vi "RGB WS2812 Control VI_DYLAN_DONE0312_Computertime.vi"() -> ()   [LabVIEW 2019]
uses:
  VI States.ctl
  <vilib>/Instr/_visa.llb/VISA Configure Serial Port (Instr).vi
  <vilib>/MakerHub/LINX/LMH-LINX.lvlib
panel:
  in  "OK Button":bool
  in  "RED 3":dbl(slide) scale=0.0..250.0
  out "RED 4":dbl format="%#_3g"
  in  "?":dbl(slide) scale=0.0..250.0
  out "?":dbl format="%#_3g"
  in  "OK Button 2":bool
  in  "Black [s]":i32
  in  "Blue [s]":i32
  in  "Red [s]":u32
  out "BlueLED":bool
  out "RedLED":bool
  out "Current date string":string
  out "Current time string":string
  out "Start light":bool
  in  "Set time x:xx AM format 2":string="8:55 AM"
  in  "VISA resource name":refnum<visa-resource-name>
  in  "Stop Button":bool
  out "Loop \nRate (Hz)":u32
  out "LeftY 2":i32
  out "LeftX 2":i32
  in  "To 1st left = dont touch":dbl format="%#_13g"
  in  "Set time x:xx AM format":string="8:55 AM"
  out "x = y?":bool
  out "time string":string
  out "date string":string
  in  "stop 2":bool
  out "Walking":bool
  in  "GO":bool
  out "RightY":i32
  out "LeftY":i32
  out "RightX":i32
  out "LeftX":i32
  in  "Repeats":i32
  in  "To Right [s]":dbl format="%#_13g"
  in  "To Left[s]":dbl format="%#_13g"
  in  "PyModule for Python 3.7":path=path "C:/Users/xwghu/Desktop/AutoControlKit/mouseControl.py"
  out "?":refnum<k35>
  in  "Python version":string="3.7"
  # "Mouse control"
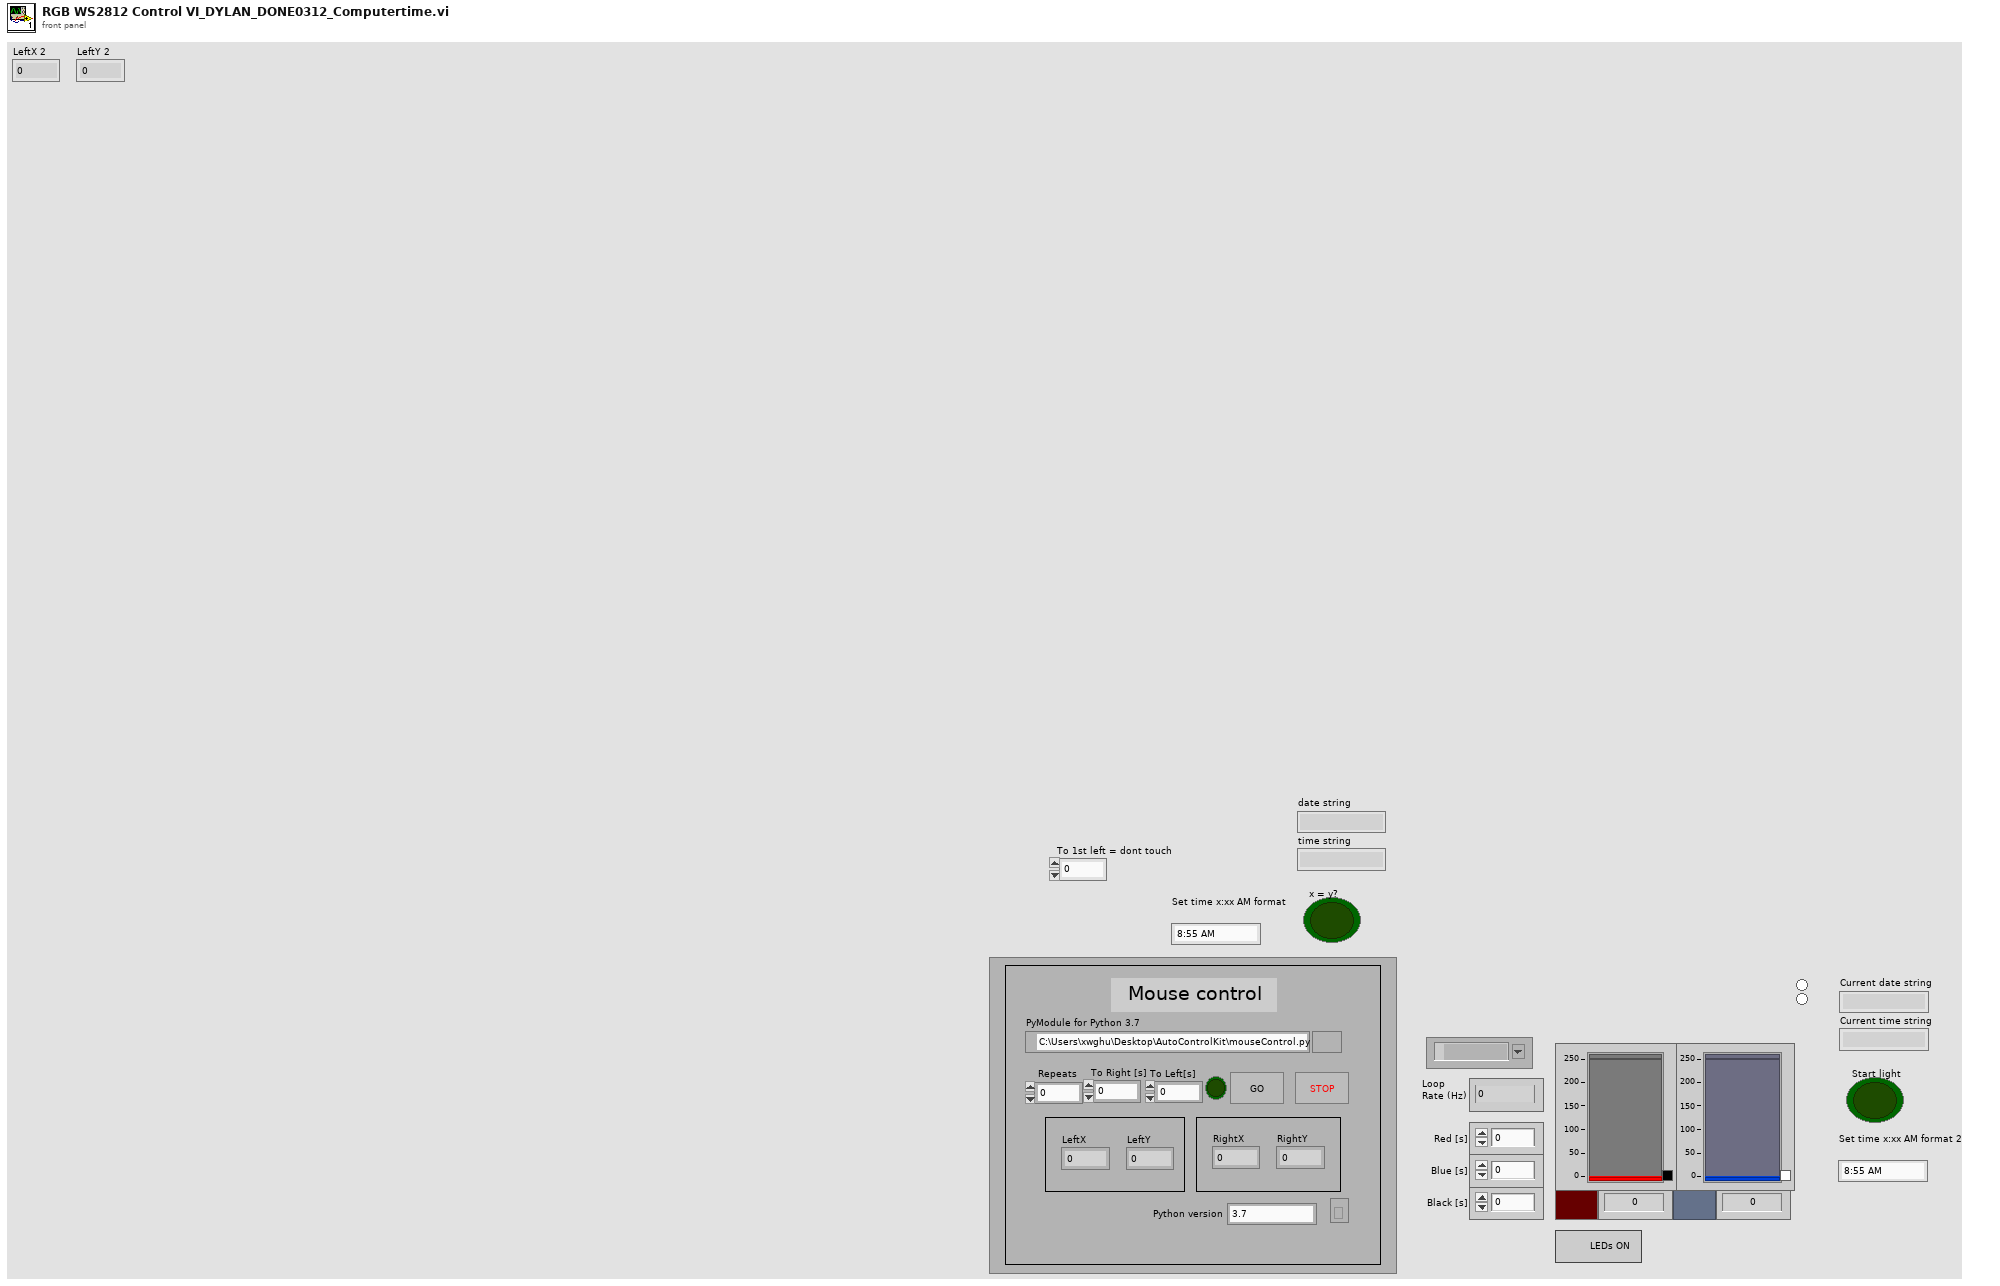
[diagram p1: front panel]
types:
  T1 = typedef "VI States.ctl" = enum16{"Poll", "Init Serial", "Read Serial", "Acq Sound", "Close Serial"}
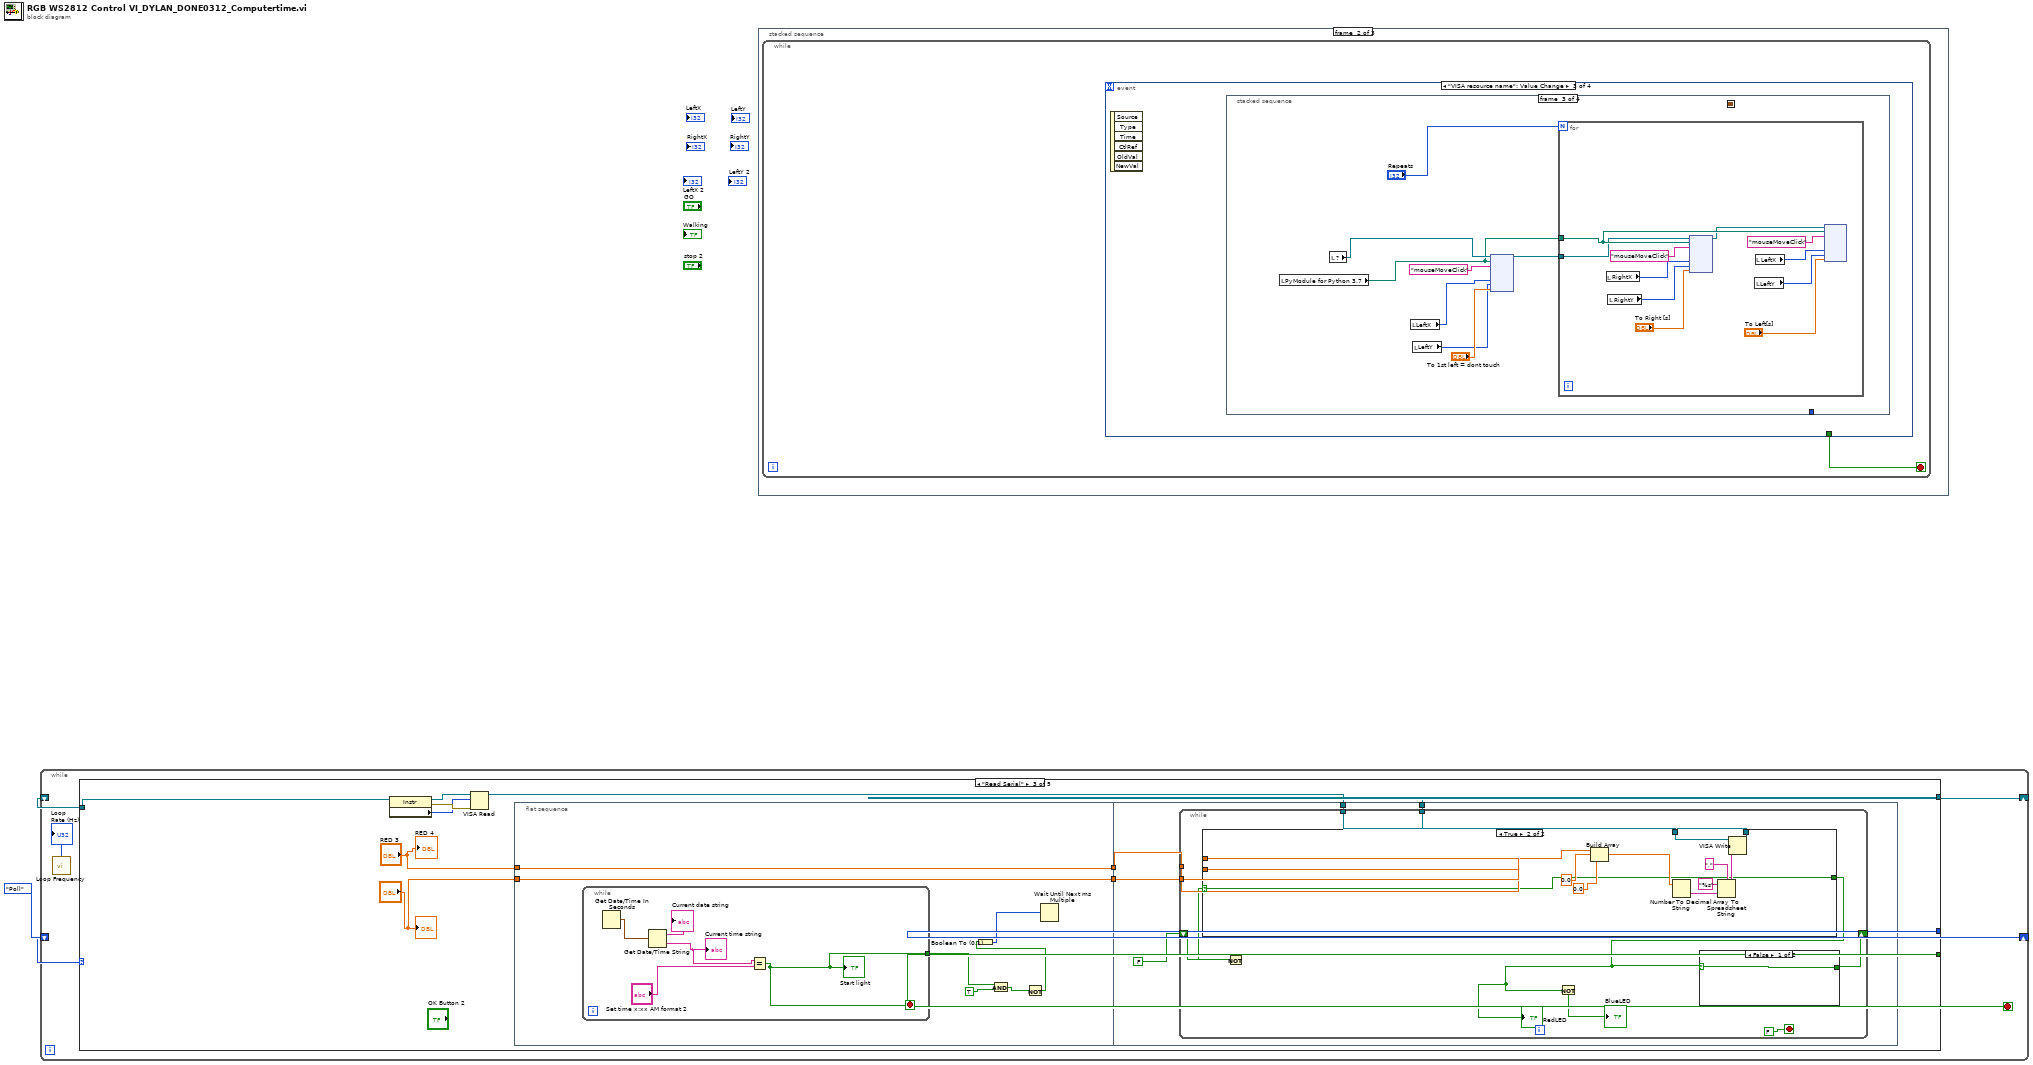
[diagram p0: block diagram]
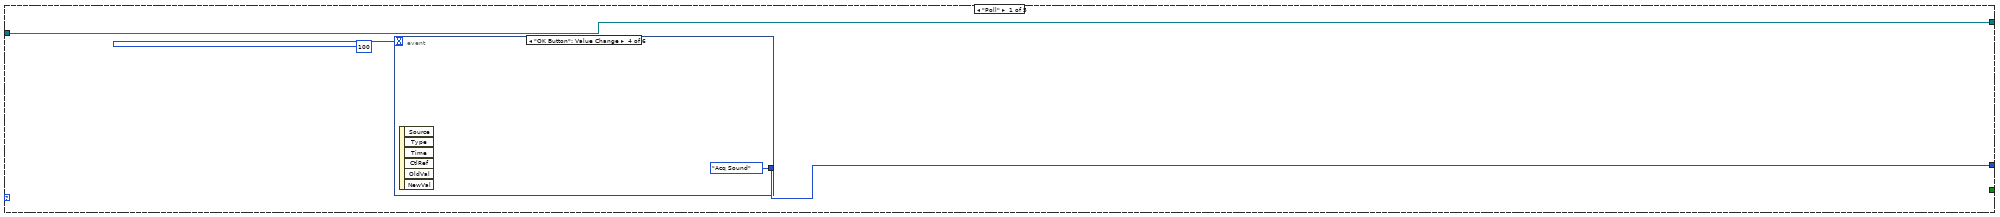
[diagram p2: hidden frame]
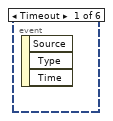
[diagram p3: hidden frame]
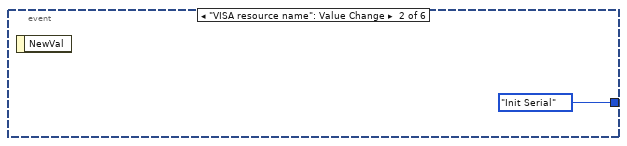
[diagram p4: hidden frame]
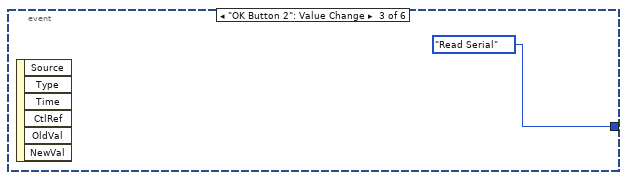
[diagram p5: hidden frame]
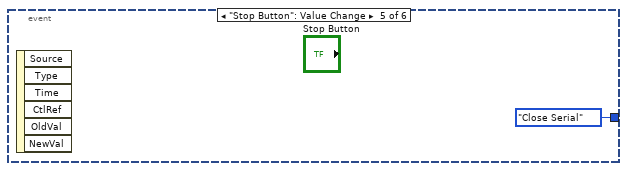
[diagram p6: hidden frame]
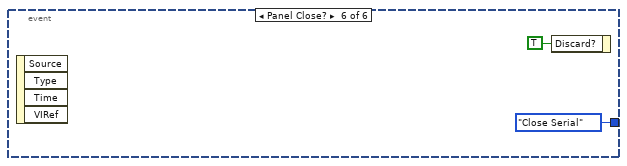
[diagram p7: hidden frame]
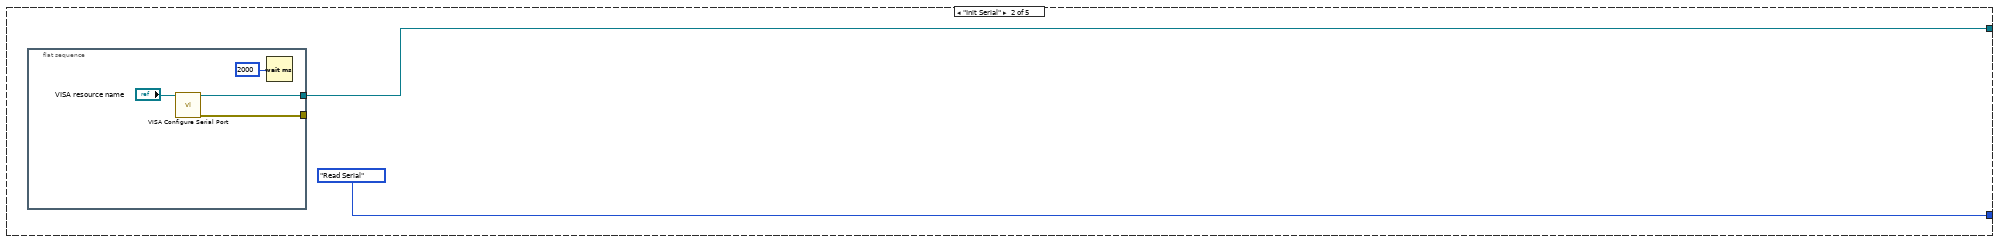
[diagram p8: hidden frame]
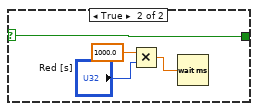
[diagram p9: hidden frame]
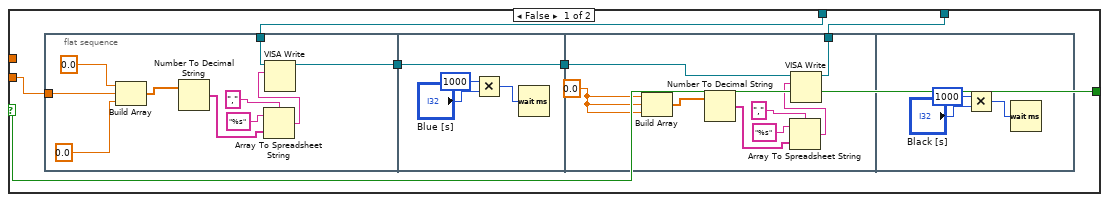
[diagram p10: hidden frame]
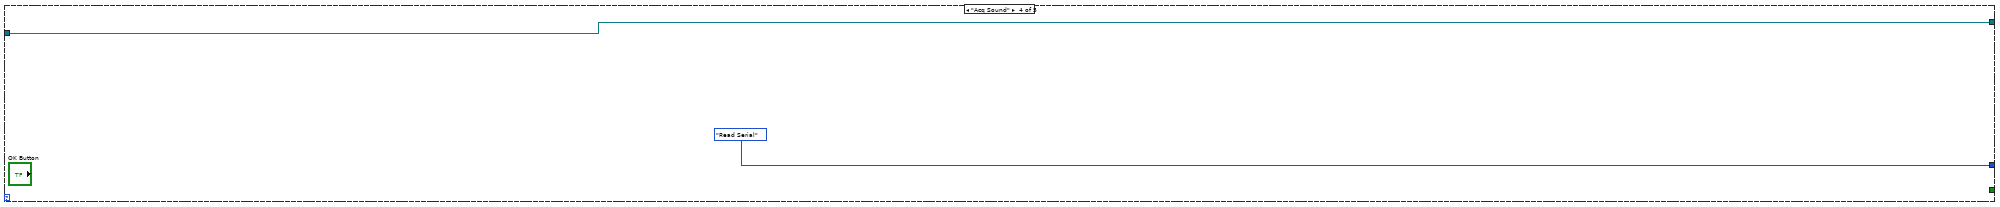
[diagram p11: hidden frame]
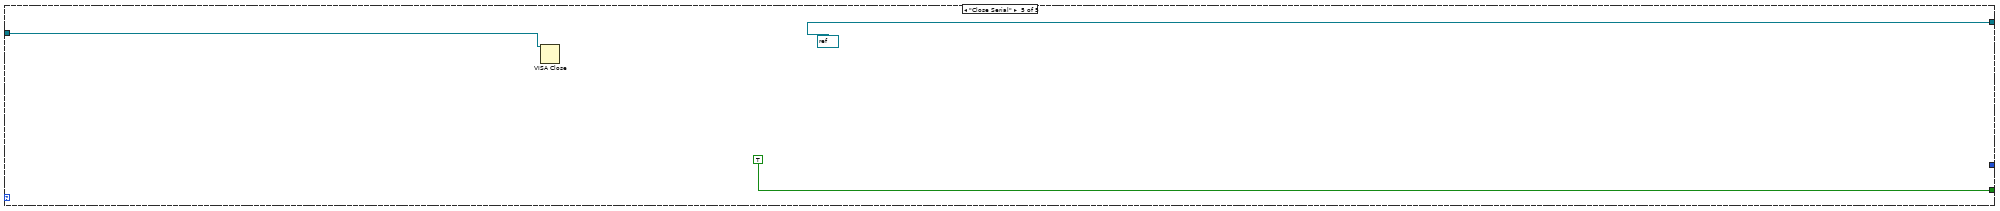
[diagram p12: hidden frame]
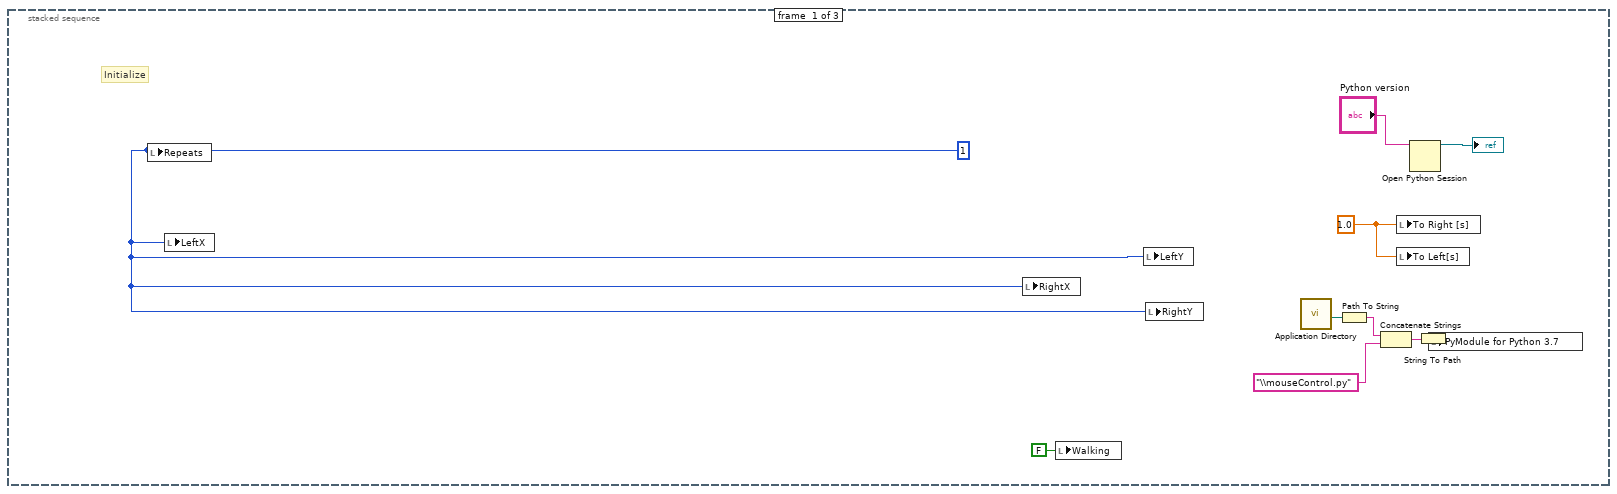
[diagram p13: hidden frame]
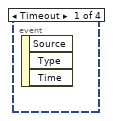
[diagram p14: hidden frame]
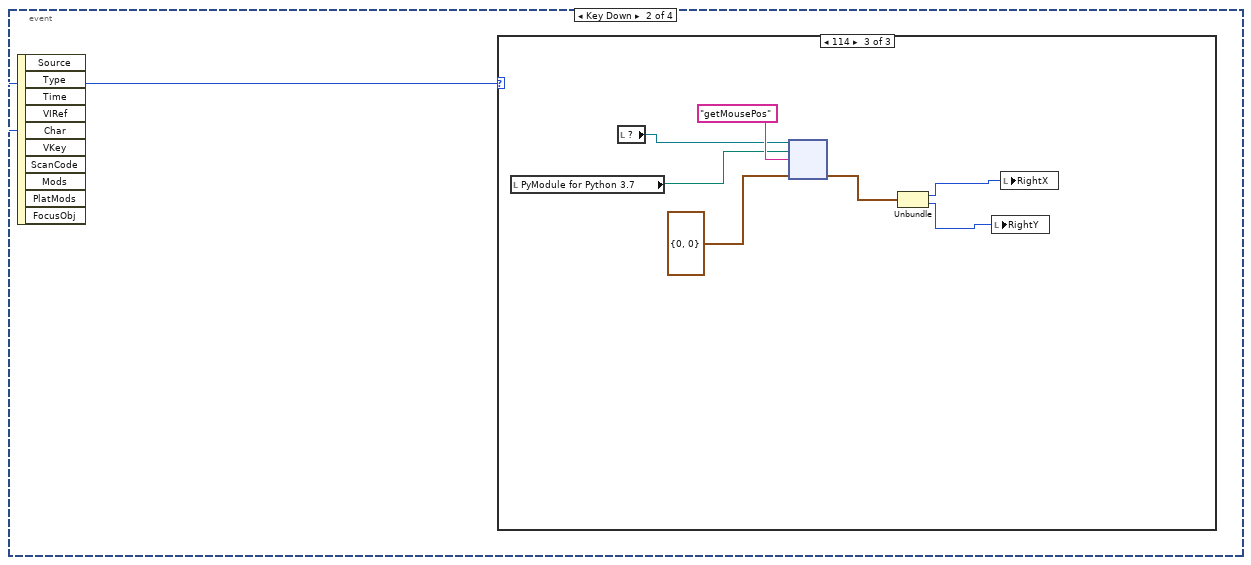
[diagram p15: hidden frame]
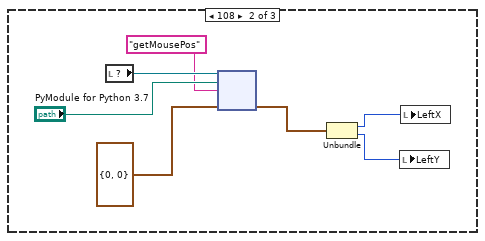
[diagram p17: hidden frame]
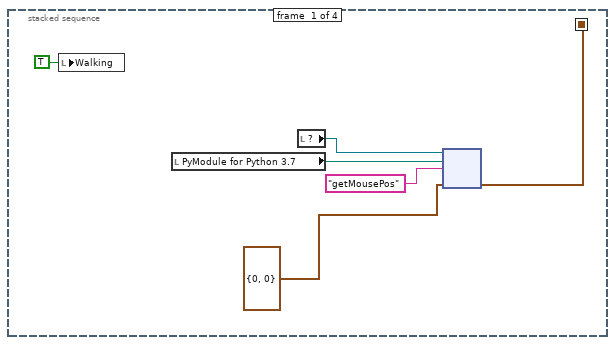
[diagram p18: hidden frame]
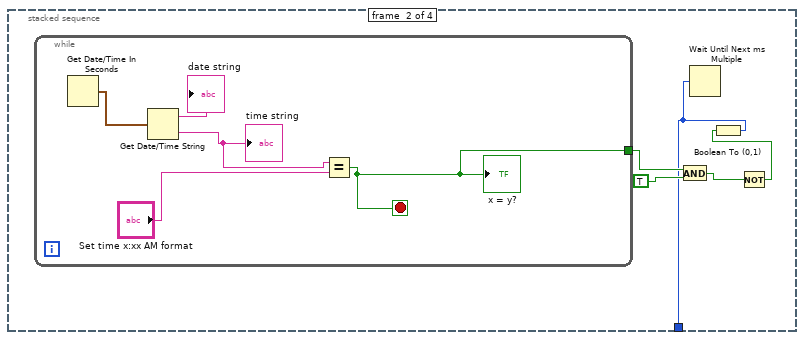
[diagram p19: hidden frame]
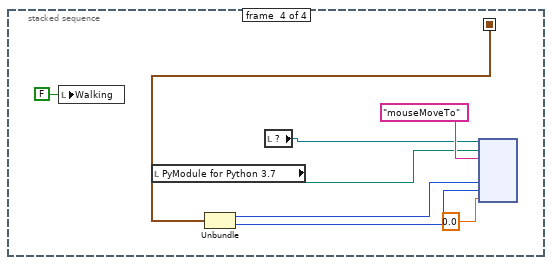
[diagram p20: hidden frame]
diagram:
  n1 = while {
    shift-right: [w6] -> _
    shift-left: VI_States."Poll" -> [w7]
    shift-right: [w2] -> _
    shift-left: _ -> [w5]
    stop <- w4 stop-if-true
    n2 = call <vilib>:"Loop Frequency.vi"() -> ("Loop Rate (Hz)"=→"Loop \nRate (Hz)":u32)
    n3 = case shown="\"Read Serial\"" w7 {
      tunnel: [w9 VI_States."Read Serial" _ VI_States."Read Serial" _] -> w6
      tunnel: [w8 w18 w27 w107 refnum<visa-resource-name> refnum ("VISA resource name out")] -> w2
      tunnel: w5 -> [w8 _ w29 w107 w111]
      tunnel: [_ _ _ _ TRUE ("Boolean")] -> w4
      frame "Poll" {
        n4 = event shown="[3] \"OK Button\": Value Change" {
          selector: _ -> [_ _ _ _ _ _]
          dyn-events: _ -> [_ _ _ _ _ _]
          timeout: 100 -> [_ _ _ _ _ _]
          tunnel: [_ VI_States."Init Serial" VI_States."Read Serial" VI_States."Acq Sound" VI_States."Close Serial" VI_States."Close Serial"] -> w9
          event Timeout {
            n5 = event-data() -> ()  [unwired: 1 in, 3 out]
          }
          event "VISA resource name": Value Change {
            n6 = event-data() -> ()  [unwired: 1 in, 1 out]
          }
          event "OK Button 2": Value Change {
            n7 = event-data() -> ()  [unwired: 1 in, 6 out]
          }
          event "OK Button": Value Change {
            n8 = event-data() -> ()  [unwired: 1 in, 6 out]
          }
          event "Stop Button": Value Change {
            n9 = event-data() -> ()  [unwired: 1 in, 6 out]
          }
          event Panel Close? {
            n10 = event-data() -> ()  [unwired: 1 in, 4 out]
            n11 = event-data("Discard?"=TRUE) -> ()  [unwired: 1 in, 1 out]
          }
        }
      }
      frame "Init Serial" {
        n12 = flat-sequence {
          tunnel: [w22] -> w18
          tunnel: [w21] -> _
          frame #0 {
            n13 = call-poly "VISA Configure Serial Port"("VISA resource name"="VISA resource name") -> ("VISA resource name out"=w22:refnum<visa-resource-name>, "error out"=w21:errorcluster)  [unwired: 8 in, 5 out]
            n14 = Wait (ms)(milliseconds to wait=u32 2000) -> ()  [unwired: 1 out]
          }
        }
      }
      frame "Read Serial" {
        n15 = property class="Instr"(reference=w29) -> (reference out=w32:refnum<visa-resource-name>, error out=w31:errorcluster, "Serial Settings:Number of Bytes at Serial Port"=w30:u32)  [unwired: 1 in]
        n16 = VISA Read(VISA resource name=w32, byte count=w30, error in (no error)=w31) -> (VISA resource name out=w28:refnum<visa-resource-name>)  [unwired: 3 out]
        n17 = flat-sequence {
          tunnel: "?" -> [w38]
          tunnel: "RED 3" -> [w39]
          tunnel: [w39] -> w24
          tunnel: [w38] -> w23
          tunnel: w28 -> [w48]
          tunnel: [w47] -> w27
          tunnel: w24 -> [w46]
          tunnel: w23 -> [w45]
          frame #0 {
            n18 = while {
              tunnel: [w40] -> w37
              stop <- w40 stop-if-true
              n19 = Get Date/Time In Seconds() -> (seconds since 1Jan1904=w44:timestamp)
              n20 = Get Date/Time String(seconds (now)=w44) -> (date string=→"Current date string":string, time string=w42:string)  [unwired: 2 in]
              "Current time string" <- w42
              n21 = Equal?(x=w42, y="Set time x:xx AM format 2") -> (x = y?=w40:bool)
              "Start light" <- w40
            }
            n22 = And(x=w37, y=TRUE) -> (x .and. y?=w35:bool)
            n23 = Not(x=w35) -> (.not. x?=w34:bool)
            n24 = Boolean To (0,1)(Boolean=w34) -> (0, 1=w33:i16)
            n25 = Wait Until Next ms Multiple(millisecond multiple=w33) -> ()  [unwired: 1 out]
          }
          frame #1 {
            n26 = while {
              shift-right: [w52] -> _
              shift-left: FALSE -> [w59]
              tunnel: w48 -> [w58]
              tunnel: [w57] -> w47
              tunnel: w46 -> [w55]
              tunnel: w45 -> [w54]
              stop <- FALSE stop-if-true
              n27 = Not(x=w59) -> (.not. x?=w53:bool)
              n28 = case shown="True" w53 {
                selector: w53 -> [w70 w96]
                tunnel: [w70 w96] -> w50
                tunnel: w58 -> [w68 w100]
                tunnel: [w65 w99] -> w57
                tunnel: w55 -> [_ w97]
                tunnel: w54 -> [w69 _]
                frame False {
                  n29 = flat-sequence {
                    tunnel: w69 -> [w73]
                    tunnel: w68 -> [w72]
                    tunnel: [w71] -> w66
                    tunnel: [w81] -> w67
                    tunnel: w66 -> [w81]
                    tunnel: w67 -> [w86]
                    tunnel: [w85] -> w65
                    frame #0 {
                      n30 = Build Array(0.0 ("element"), w73, 0.0 ("element")) -> (w76:dbl[])
                      n31 = Number To Decimal String(number=w76) -> (decimal integer string=w77:string[])  [unwired: 1 in]
                      n32 = Array To Spreadsheet String(delimiter (Tab)=",", array=w77, 3:"%s" ("format string")) -> (spreadsheet string=w80:string)
                      n33 = VISA Write(VISA resource name=w72, write buffer=w80) -> (VISA resource name out=w71:refnum<visa-resource-name>)  [unwired: 1 in, 2 out]
                    }
                    frame #1 {
                      n34 = Multiply(x=1000, y="Blue [s]") -> (x*y=w82:i32)
                      n35 = Wait (ms)(milliseconds to wait=w82) -> ()  [unwired: 1 out]
                    }
                    frame #2 {
                      w87 = 0.0 ("element")
                      n36 = Build Array(w87, w87, w87) -> (w88:dbl[])
                      n37 = Number To Decimal String(number=w88) -> (decimal integer string=w89:string[])  [unwired: 1 in]
                      n38 = Array To Spreadsheet String(delimiter (Tab)=",", array=w89, 3:"%s" ("format string")) -> (spreadsheet string=w92:string)
                      n39 = VISA Write(VISA resource name=w86, write buffer=w92) -> (VISA resource name out=w85:refnum<visa-resource-name>)  [unwired: 1 in, 2 out]
                    }
                    frame #3 {
                      n40 = Multiply(x=1000, y="Black [s]") -> (x*y=w93:i32)
                      n41 = Wait (ms)(milliseconds to wait=w93) -> ()  [unwired: 1 out]
                    }
                  }
                }
                frame True {
                  n42 = Build Array(w97, 0.0 ("element"), 0.0 ("element")) -> (w98:dbl[])
                  n43 = Number To Decimal String(number=w98) -> (decimal integer string=w104:string[])  [unwired: 1 in]
                  n44 = Array To Spreadsheet String(delimiter (Tab)=",", array=w104, 3:"%s" ("format string")) -> (spreadsheet string=w103:string)
                  n45 = VISA Write(VISA resource name=w100, write buffer=w103) -> (VISA resource name out=w99:refnum<visa-resource-name>)  [unwired: 1 in, 2 out]
                }
              }
              "RedLED" <- w50
              n46 = Not(x=w50) -> (.not. x?=→"BlueLED":bool)
              n47 = case shown="False" w50 {
                selector: w50 -> [w60 w64]
                tunnel: [w60 w64] -> w52
                frame False {
                }
                frame True {
                  n48 = Multiply(x=1000.0, y="Red [s]") -> (x*y=w62:dbl)
                  n49 = Wait (ms)(milliseconds to wait=w62) -> ()  [unwired: 1 out]
                }
              }
            }
          }
        }
        "RED 4" <- "RED 3"
        "?" <- "?"
      }
      frame "Acq Sound" {
      }
      frame "Close Serial" {
        n50 = VISA Close(VISA resource name=w111) -> ()  [unwired: 1 in, 1 out]
      }
    }
  }
  n51 = stacked-sequence {
    frame #0 {
      w112 = 1.0
      w113 = 1
      # "Initialize"
      n52 = local write "Repeats"(w113) -> ()
      n53 = local write "LeftX"(w113) -> ()
      n54 = local write "RightX"(w113) -> ()
      n55 = local write "Walking"(FALSE ("Walking")) -> ()
      n56 = local write "LeftY"(w113) -> ()
      n57 = local write "RightY"(w113) -> ()
      n58 = call <vilib>:"Application Directory.vi"() -> ("Application Directory"=w118:path)
      n59 = Path To String(path=w118) -> (string=w117:string)
      n60 = Concatenate Strings(w117, "\\mouseControl.py") -> (w115:string)
      n61 = local write "To Right [s]"(w112) -> ()
      n62 = local write "To Left[s]"(w112) -> ()
      n63 = Open Python Session(python version="Python version") -> (session out=→"?":refnum<k35>)  [unwired: 2 in, 1 out]
      n64 = String To Path(string=w115) -> (path=w114:path)
      n65 = local write "PyModule for Python 3.7"(w114) -> ()
    }
    frame #1 {
      n66 = while {
        stop <- w122 stop-if-true
        n67 = event shown="[2] \"VISA resource name\": Value Change" {
          selector: _ -> [_ _ _ _]
          dyn-events: _ -> [_ _ _ _]
          timeout: _ -> [_ _ _ _]
          tunnel: [_ _ _ TRUE] -> w122
          event Timeout {
            n68 = event-data() -> ()  [unwired: 1 in, 3 out]
          }
          event Key Down {
            n69 = event-data() -> ("Char"=w123:i16)  [unwired: 1 in, 9 out]
            n70 = case shown="114" w123 {
              frame 0, Default {
              }
              frame 108 {
                n71 = local read item#1() -> (w130:refnum<k35>)
                n72 = node(w130, "PyModule for Python 3.7", "getMousePos" ("function name"), cluster{i32, i32} {0, 0}) -> (w126:cluster{i32, i32})  [unwired: 1 in, 4 out]
                n73 = Unbundle(w126) -> (w125:i32, w124:i32)
                n74 = local write "LeftY"(w124) -> ()
                n75 = local write "LeftX"(w125) -> ()
              }
              frame 114 {
                n76 = local read "PyModule for Python 3.7"() -> (w133:path)
                n77 = local read item#1() -> (w134:refnum<k35>)
                n78 = node(w134, w133, "getMousePos" ("function name"), cluster{i32, i32} {0, 0}) -> (w135:cluster{i32, i32})  [unwired: 1 in, 4 out]
                n79 = Unbundle(w135) -> (w131:i32, w132:i32)
                n80 = local write "RightY"(w132) -> ()
                n81 = local write "RightX"(w131) -> ()
              }
            }
          }
          event "VISA resource name": Value Change {
            n82 = event-data() -> ()  [unwired: 1 in, 6 out]
            n83 = stacked-sequence {
              seq-local: [w138 _ _ _] -> [_ _ _ w175]
              tunnel: [_ w144 _ _] -> _
              frame #0 {
                n84 = local write "Walking"(TRUE ("Walking")) -> ()
                n85 = local read "PyModule for Python 3.7"() -> (w141:path)
                n86 = local read item#1() -> (w142:refnum<k35>)
                n87 = node(w142, w141, "getMousePos" ("function name"), cluster{i32, i32} {0, 0}) -> (w138:cluster{i32, i32})  [unwired: 1 in, 4 out]
              }
              frame #1 {
                n88 = while {
                  tunnel: [w149] -> w148
                  stop <- w149 stop-if-true
                  n89 = Get Date/Time In Seconds() -> (seconds since 1Jan1904=w153:timestamp)
                  n90 = Get Date/Time String(seconds (now)=w153) -> (date string=→"date string":string, time string=w151:string)  [unwired: 2 in]
                  "time string" <- w151
                  n91 = Equal?(x=w151, y="Set time x:xx AM format") -> (x = y?=w149:bool)
                  "x = y?" <- w149
                }
                n92 = And(x=w148, y=TRUE) -> (x .and. y?=w146:bool)
                n93 = Not(x=w146) -> (.not. x?=w145:bool)
                n94 = Boolean To (0,1)(Boolean=w145) -> (0, 1=w144:i16)
                n95 = Wait Until Next ms Multiple(millisecond multiple=w144) -> ()  [unwired: 1 out]
              }
              frame #2 {
                n96 = local read "PyModule for Python 3.7"() -> (w155:path)
                n97 = local read item#1() -> (w160:refnum<k35>)
                n98 = local read "LeftX"() -> (w157:i32)
                n99 = local read "LeftY"() -> (w156:i32)
                n100 = node(w160, w155, "mouseMoveClick" ("function name"), w157, w156, "To 1st left = dont touch") -> (w154:refnum<k35>)  [unwired: 6 in, 3 out]
                n101 = for {
                  N: "Repeats" -> [_]
                  tunnel: w155 -> [w164]
                  tunnel: w154 -> [w163]
                  n102 = local read "RightX"() -> (w171:i32)
                  n103 = local read "RightY"() -> (w170:i32)
                  n104 = node(w163, w164, "mouseMoveClick" ("function name"), w171, w170, "To Right [s]") -> (w162:refnum<k35>)  [unwired: 6 in, 3 out]
                  n105 = local read "LeftY"() -> (w167:i32)
                  n106 = local read "LeftX"() -> (w168:i32)
                  n107 = node(w162, w164, "mouseMoveClick" ("function name"), w168, w167, "To Left[s]") -> ()  [unwired: 6 in, 4 out]
                }
              }
              frame #3 {
                n108 = local write "Walking"(FALSE ("Walking")) -> ()
                n109 = local read "PyModule for Python 3.7"() -> (w176:path)
                n110 = Unbundle(w175) -> (w174:i32, w173:i32)
                n111 = local read item#1() -> (w177:refnum<k35>)
                n112 = node(w177, w176, "mouseMoveTo" ("function name"), w174, w173, 0.0) -> ()  [unwired: 6 in, 4 out]
              }
            }
          }
          event "stop 2": Mouse Up {
            n113 = event-data() -> ()  [unwired: 1 in, 8 out]
          }
        }
      }
    }
    frame #2 {
      n114 = local read item#1() -> (w182:refnum<k35>)
      n115 = Close Python Session(session in=w182) -> ()  [unwired: 1 in, 1 out]
    }
  }
